vi "ep_Load Check Error (N Chan).vi"(1 "additional efficiency information":T1(array[cluster]), 7 "speed [RPM]":dbl[](array[numeric]), 9 "nameplate information":T2(array[cluster]), 11 "error in (no error)":errorcluster, 12 "total input active power [W]":dbl[](array[numeric])) -> (2 "number of motors":i32, 3 "non-empty speed?":bool, 15 "error out":errorcluster)   [LabVIEW 2014, in "NI_EP_Motor Monitoring.lvlib"]
uses:
  <vilib>/addons/Electrical Power/Motor Monitoring/NI_EP_Motor Monitoring.lvlib
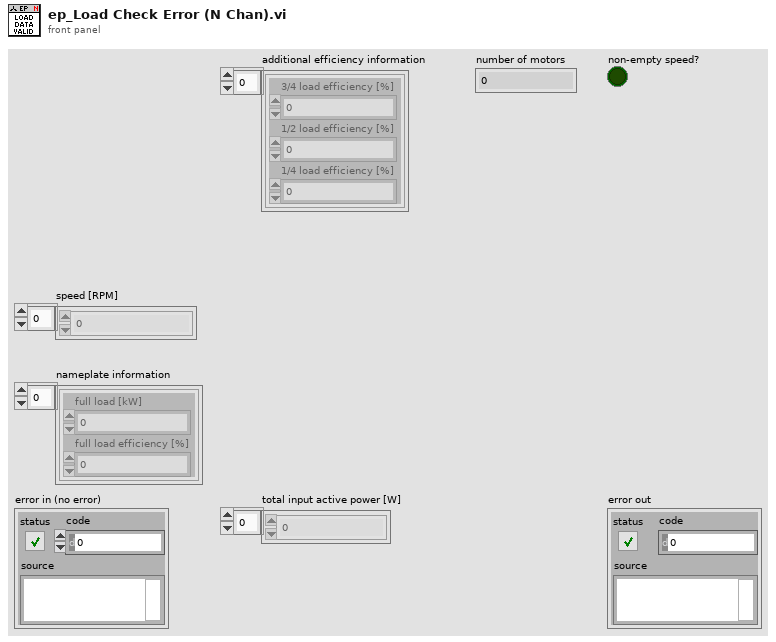
[diagram p1: front panel]
types:
  T1 = cluster{"3/4 load efficiency [%]":dbl, "1/2 load efficiency [%]":dbl, "1/4 load efficiency [%]":dbl}[]
  T2 = cluster{"full load [kW]":dbl, "full load efficiency [%]":dbl}[]
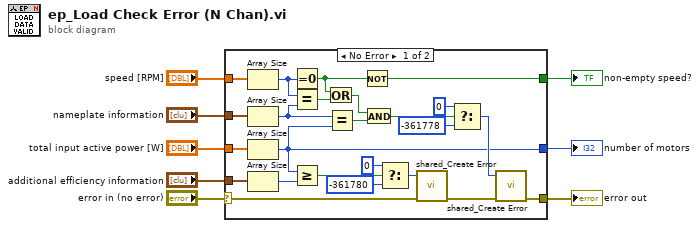
[diagram p0: block diagram]
diagram:
  n1 = case shown="No Error" "error in (no error)" {
    selector: "error in (no error)" -> [w26 w33]
    tunnel: [w22 w33] -> w7
    tunnel: "total input active power [W]" -> [w32 _]
    tunnel: "nameplate information" -> [w31 _]
    tunnel: "speed [RPM]" -> [w30 _]
    tunnel: "additional efficiency information" -> [w29 _]
    tunnel: [w12 _] -> w3
    tunnel: [w9 _] -> w1
    frame No Error {
      n2 = Array Size(array=w30) -> (size(s)=w20:i32)
      n3 = Array Size(array=w31) -> (size(s)=w19:i32)
      n4 = Array Size(array=w32) -> (size(s)=w12:i32)
      n5 = Array Size(array=w29) -> (size(s)=w13:i32)
      n6 = Equal To 0?(x=w20) -> (x = 0?=w10:bool)
      n7 = Equal?(x=w20, y=w19) -> (x = y?=w18:bool)
      n8 = Greater Or Equal?(x=w12, y=w13) -> (x >= y?=w21:bool)
      n9 = Or(x=w10, y=w18) -> (x .or. y?=w16:bool)
      n10 = Equal?(x=w19, y=w12) -> (x = y?=w17:bool)
      n11 = Not(x=w10) -> (.not. x?=w9:bool)
      n12 = And(x=w16, y=w17) -> (x .and. y?=w11:bool)
      n13 = Select(t=0, s=w21, f=-361780) -> (s? t:f=w15:i32)
      n14 = call <vilib>:"shared_Create Error.vi"("error in (no error)"=w26, "error code (0)"=w15) -> ("error out"=w23:errorcluster)  [unwired: 9 in]
      n15 = Select(t=0, s=w11, f=-361778) -> (s? t:f=w14:i32)
      n16 = call <vilib>:"shared_Create Error.vi"("error in (no error)"=w23, "error code (0)"=w14) -> ("error out"=w22:errorcluster)  [unwired: 9 in]
    }
    frame Error {
    }
  }
  "error out" <- w7
  "number of motors" <- w3
  "non-empty speed?" <- w1
